vi "Temperature Limit.vi"() -> ()   [LabVIEW 2015]
doc: "This VI simulates the acquisition of temperature, graphs the temperature, and notifies the user if the temperature is over the limit."
panel:
  in  "Start":bool
  in  "Delta t (ms)":i32(slide)=400 scale=50.0..500.0
  in  "Stop":bool
  in  "High Limit":dbl=28.0 format="%.2f"
  out "Temperature":cluster{"Temperature":dbl, "High Limit":dbl}(graph)={"Temperature"=85.88749999999999, "High Limit"=80.0}
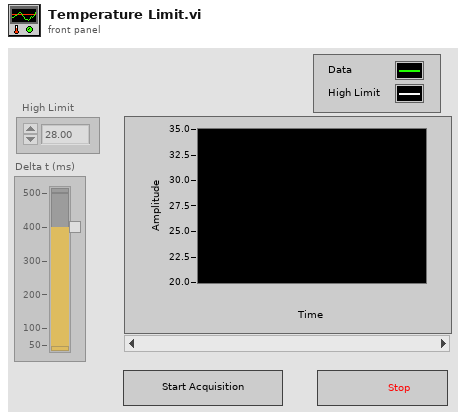
[diagram p1: front panel]
types:
  T1 = enum8{"Enabled", "Disabled", "Disabled and Grayed Out"}
  T2 = cluster{"Temperature Value":dbl, "High Limit":dbl}
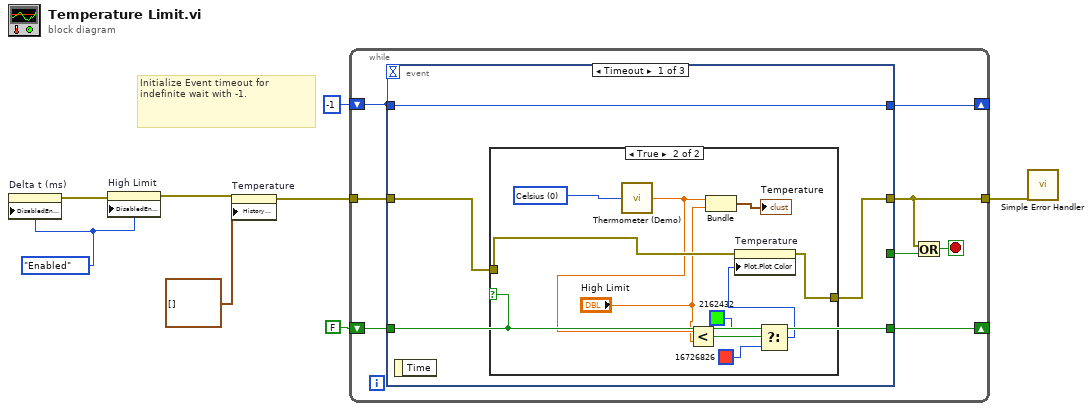
[diagram p0: block diagram]
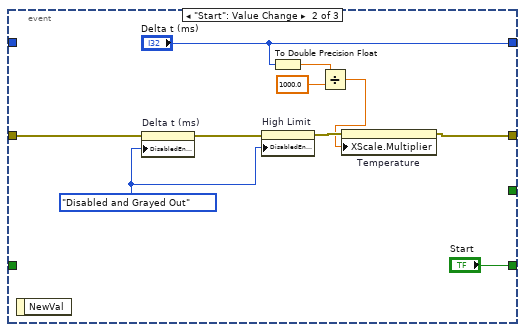
[diagram p3: hidden frame]
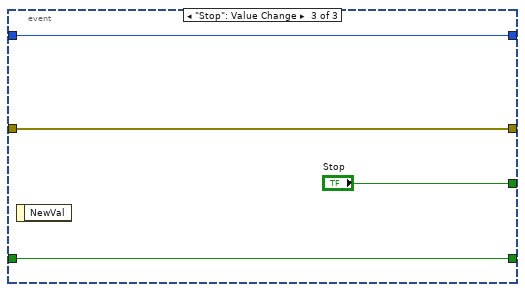
[diagram p4: hidden frame]
diagram:
  w5 = T1."Enabled" ("Disabled")
  # "Initialize Event timeout for indefinite wait with -1."
  n1 = property on="Delta t (ms)" class="Slide (strict)"("DisabledEnum"=w5) -> (error out=w4:errorcluster)  [unwired: 2 in, 1 out]
  n2 = property on="High Limit" class="DigNum (strict)"(error in=w4, "DisabledEnum"=w5) -> (error out=w2:errorcluster)  [unwired: 1 in, 1 out]
  n3 = property on="Temperature" class="WFChart (strict)"(error in=w2, "History Data"=cluster{"Temperature":dbl, "High Limit":dbl}[] []) -> (error out=w1:errorcluster)  [unwired: 1 in, 1 out]
  n4 = while {
    tunnel: w1 -> [w16]
    tunnel: [w14] -> w7
    shift-right: [w12] -> _
    shift-left: FALSE ("Start") -> [w11]
    shift-right: [w10] -> _
    shift-left: -1 ("Delta t (ms)") -> [w9]
    stop <- w15 stop-if-true
    n5 = event shown="[0] Timeout" {
      selector: _ -> [_ _ _]
      dyn-events: _ -> [_ _ _]
      timeout: w9 -> [_ _ _]
      tunnel: [_ _ "Stop"] -> w13
      tunnel: w16 -> [w18 w39 w43]
      tunnel: [w17 w36 w43] -> w14
      tunnel: [w19 "Start" w42] -> w12
      tunnel: w11 -> [w19 _ w42]
      tunnel: [w20 "Delta t (ms)" w41] -> w10
      tunnel: w9 -> [w20 _ w41]
      event Timeout {
        n6 = event-data() -> ()  [unwired: 1 in, 1 out]
        n7 = case shown="True" w19 {
          tunnel: w18 -> [_ w28]
          tunnel: [_ w27] -> w17
          frame False {
          }
          frame True {
            w29 = u16 0 items=["Celsius", "Fahrenheit"] ("Units (0: Celsius)")
            n8 = call "Thermometer (Demo).vi"("Units (0: Celsius)"=w29) -> ("Temperature Value"=w26:dbl)
            n9 = Less?(x=w26, y="High Limit") -> (x < y?=w21:bool)
            n10 = Bundle("Temperature Value"=w26, "High Limit"="High Limit") -> (→"Temperature":T2)  [unwired: 1 in]
            n11 = Select(t=u32 2162432, s=w21, f=u32 16726826) -> (s? t:f=w22:u32)
            n12 = property on="Temperature" class="WFChart (strict)"(error in=w28, "Plot.Plot Color"=w22) -> (error out=w27:errorcluster)  [unwired: 1 in, 1 out]
          }
        }
      }
      event "Start": Value Change {
        w31 = T1."Disabled and Grayed Out" ("Disabled")
        n13 = event-data() -> ()  [unwired: 1 in, 1 out]
        n14 = property on="Delta t (ms)" class="Slide (strict)"(error in=w39, "DisabledEnum"=w31) -> (error out=w38:errorcluster)  [unwired: 1 in, 1 out]
        n15 = property on="High Limit" class="DigNum (strict)"(error in=w38, "DisabledEnum"=w31) -> (error out=w37:errorcluster)  [unwired: 1 in, 1 out]
        n16 = To Double Precision Float(number="Delta t (ms)") -> (double precision float=w34:dbl)
        n17 = Divide(x=w34, y=1000.0) -> (x/y=w33:dbl)
        n18 = property on="Temperature" class="WFChart (strict)"(error in=w37, "XScale.Multiplier"=w33) -> (error out=w36:errorcluster)  [unwired: 1 in, 1 out]
      }
      event "Stop": Value Change {
        n19 = event-data() -> ()  [unwired: 1 in, 1 out]
      }
    }
    n20 = Or(x=w14, y=w13) -> (x .or. y?=w15:bool)
  }
  n21 = call <vilib>:"Simple Error Handler.vi"("error in (no error)"=w7) -> ()  [unwired: 4 in, 5 out]
